vi "Write R.vi"(8 "error in (no error)":errorcluster, 10 "Real Matrix":T1, 11 "Ball in":refnum<class "Ball.lvclass">) -> (0 "error out":errorcluster, 3 "Ball out":refnum<class "Ball.lvclass">)   [LabVIEW 2018, in "Ball.lvclass"]
uses:
  Ball.lvclass
  <vilib>/Analysis/Matrix/Datatypes/RealMatrix.ctl
  Ball.lvclass/Ball.ctl
  <vilib>/Analysis/Matrix/NI_Matrix.lvlib
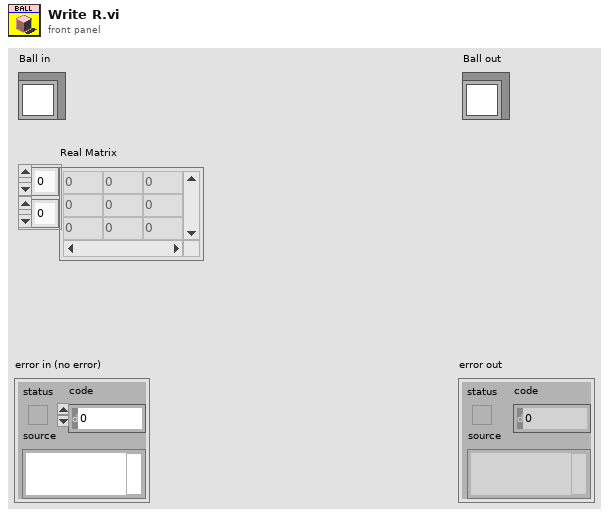
[diagram p1: front panel]
types:
  T1 = typedef "NI_Matrix.lvlib/RealMatrix.ctl" = dbl[][]
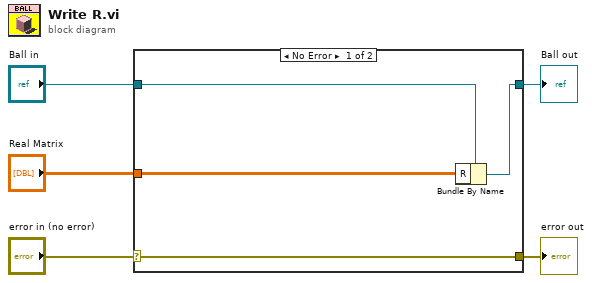
[diagram p0: block diagram]
diagram:
  n1 = case shown="No Error" "error in (no error)" {
    selector: "error in (no error)" -> [w9 w10]
    tunnel: [w9 w10] -> w4
    tunnel: [w7 w11] -> w2
    tunnel: "Ball in" -> [w8 w11]
    tunnel: "Real Matrix" -> [w6 _]
    frame No Error {
      n2 = Bundle By Name(cluster=w8, "R"=w6) -> (w7:refnum<class "Ball.lvclass">)
    }
    frame Error {
    }
  }
  "error out" <- w4
  "Ball out" <- w2
